vi "Open EXE or VI.vi"(8 "error in (no error)":errorcluster, 11 "Paths":string[](array[string])) -> (0 "error out":errorcluster)   [LabVIEW 2019, in "Control Experiment.lvclass"]
uses:
  Control Experiment.lvclass
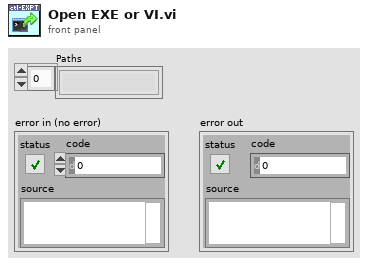
[diagram p1: front panel]
types:
  T1 = enum32{"Invalid", "Standard", "Closed", "Hidden", "Minimized", "Maximized"}
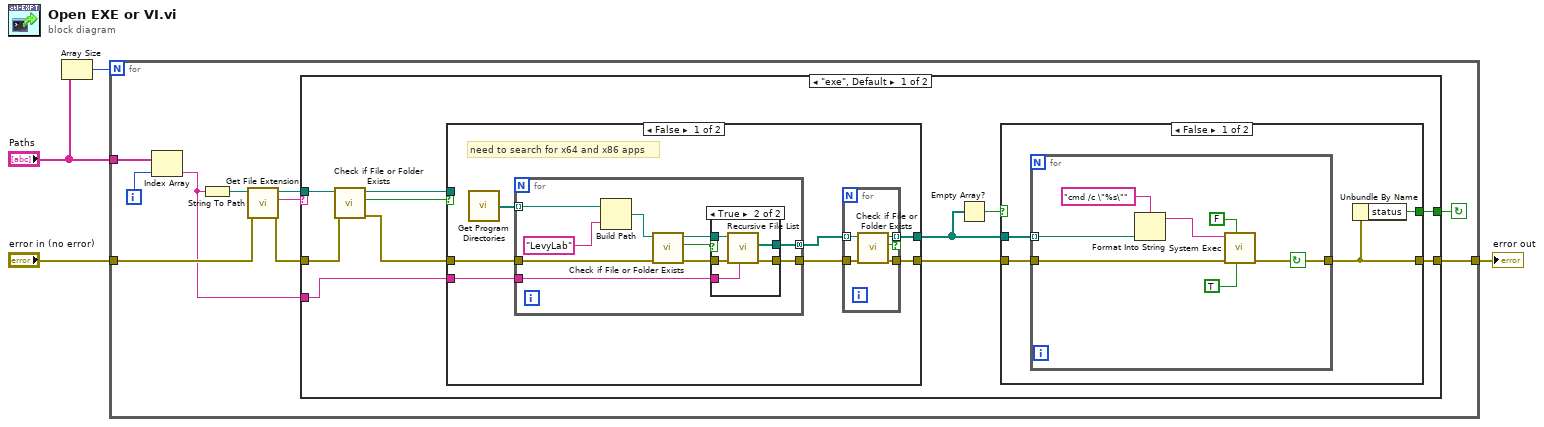
[diagram p0: block diagram]
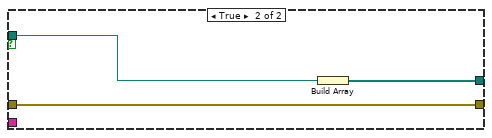
[diagram p3: hidden frame]
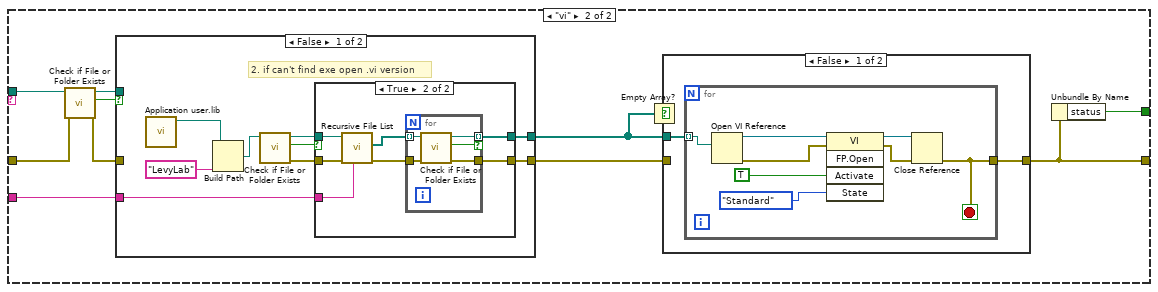
[diagram p5: hidden frame]
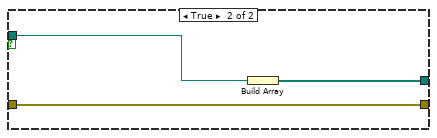
[diagram p7: hidden frame]
diagram:
  n1 = Array Size(array="Paths") -> (size(s)=w3:i32)
  n2 = for {
    N: w3 -> [_]
    tunnel: "error in (no error)" -> [w7]
    tunnel: [w14] -> w1
    tunnel: "Paths" -> [w12]
    i -> [w10]
    stop <- w13 continue-if-true
    n3 = Index Array(array=w12, index=w10) -> (element=w6:string)
    n4 = String To Path(string=w6) -> (path=w11:path)
    n5 = call <vilib>:"Get File Extension.vi"("error in (no error)"=w7, "file"=w11) -> ("error out"=w8:errorcluster, "lowercase file extension"=w9:string, "dup file"=w5:path)  [unwired: 5 in, 2 out]
    n6 = case shown="\"exe\", Default" w9 {
      tunnel: [w25 w80] -> w14
      tunnel: w8 -> [w18 w76]
      tunnel: [w23 w79] -> w13
      tunnel: w6 -> [w22 w78]
      tunnel: w5 -> [w21 w77]
      frame "exe", Default {
        n7 = call <vilib>:"Check if File or Folder Exists.vi"("error in (no error)"=w18, "path"=w21) -> ("error out"=w20:errorcluster, "file or folder exists?"=w19:bool, "dup path"=w17:path)  [unwired: 7 in]
        n8 = case shown="False" w19 {
          tunnel: w20 -> [w30 w56]
          tunnel: [w29 w56] -> w24
          tunnel: [w28 w55] -> w16
          tunnel: w22 -> [w27 _]
          tunnel: w17 -> [_ w54]
          frame False {
            # "need to search for x64 and x86 apps"
            n9 = call "Get Program Directories.vi"() -> ("Program Directories"=w32:path[])
            n10 = for {
              tunnel: w32 -> [w41] mode=indexing
              tunnel: w30 -> [w34]
              tunnel: [w40] -> w26
              tunnel: [w39] -> w31 mode=concatenating
              tunnel: w27 -> [w38]
              n11 = Build Path(base path=w41, name or relative path="LevyLab") -> (appended path=w37:path)
              n12 = call <vilib>:"Check if File or Folder Exists.vi"("error in (no error)"=w34, "path"=w37) -> ("error out"=w35:errorcluster, "file or folder exists?"=w33:bool, "dup path"=w36:path)  [unwired: 7 in]
              n13 = case shown="True" w33 {
                tunnel: [w43 w48] -> w40
                tunnel: [_ w47] -> w39
                tunnel: w38 -> [_ w46]
                tunnel: w36 -> [_ w45]
                tunnel: w35 -> [w43 w44]
                frame False {
                }
                frame True {
                  n14 = call <vilib>:"Recursive File List.vi"("pattern"=w46, "error in (no error)"=w44, "Folder Path"=w45) -> ("error out"=w48:errorcluster, "All Files in Dir"=w47:path[])  [unwired: 4 in, 3 out]
                }
              }
            }
            n15 = for {
              tunnel: w26 -> [w53]
              tunnel: w31 -> [w52] mode=indexing
              tunnel: [w51] -> w28 mode=indexing if=w49
              tunnel: [w50] -> w29
              n16 = call <vilib>:"Check if File or Folder Exists.vi"("error in (no error)"=w53, "path"=w52) -> ("error out"=w50:errorcluster, "file or folder exists?"=w49:bool, "dup path"=w51:path)  [unwired: 7 in]
            }
          }
          frame True {
            n17 = Build Array(w54) -> (w55:path[])
          }
        }
        n18 = Empty Array?(array=w16) -> (empty?=w15:bool)
        n19 = case shown="False" w15 {
          selector: w15 -> [_ w69]
          tunnel: [w58 w68] -> w25
          tunnel: w24 -> [w60 w68]
          tunnel: w16 -> [w59 _]
          tunnel: [w57 w69] -> w23
          frame False {
            n20 = for {
              tunnel: w59 -> [w62] mode=indexing
              tunnel: w60 -> [w64]
              tunnel: [w61] -> w58
              stop <- w61 continue-if-true
              n21 = Format Into String(format string="cmd /c \"%s\"", w62) -> (resulting string=w67:string)  [unwired: 2 in, 1 out]
              n22 = call <vilib>:"System Exec.vi"("run minimized? (F)"=TRUE, "wait until completion? (T)"=FALSE, "error in (no error)"=w64, "command line"=w67) -> ("error out"=w61:errorcluster)  [unwired: 4 in, 3 out]
            }
            n23 = Unbundle By Name(w58) -> ("status"=w57:bool)
          }
          frame True {
          }
        }
      }
      frame "vi" {
        n24 = call <vilib>:"Check if File or Folder Exists.vi"("error in (no error)"=w76, "path"=w77) -> ("error out"=w71:errorcluster, "file or folder exists?"=w70:bool, "dup path"=w72:path)  [unwired: 7 in]
        n25 = case shown="False" w70 {
          tunnel: [w88 w104] -> w74
          tunnel: [w87 w103] -> w73
          tunnel: w78 -> [w86 _]
          tunnel: w72 -> [_ w105]
          tunnel: w71 -> [_ w103]
          frame False {
            # "2. if can't find exe open .vi version"
            n26 = call "Application user.lib.vi"() -> ("path out"=w85:path)  [unwired: 10 in, 1 out]
            n27 = Build Path(base path=w85, name or relative path="LevyLab") -> (appended path=w84:path)
            n28 = call <vilib>:"Check if File or Folder Exists.vi"("path"=w84) -> ("error out"=w81:errorcluster, "file or folder exists?"=w82:bool, "dup path"=w83:path)  [unwired: 8 in]
            n29 = case shown="True" w82 {
              tunnel: [_ w97] -> w88
              tunnel: [w90 w96] -> w87
              tunnel: w86 -> [_ w95]
              tunnel: w83 -> [_ w93]
              tunnel: w81 -> [w90 w92]
              frame False {
              }
              frame True {
                n30 = call <vilib>:"Recursive File List.vi"("pattern"=w95, "error in (no error)"=w92, "Folder Path"=w93) -> ("error out"=w91:errorcluster, "All Files in Dir"=w94:path[])  [unwired: 4 in, 3 out]
                n31 = for {
                  tunnel: w91 -> [w102]
                  tunnel: w94 -> [w101] mode=indexing
                  tunnel: [w100] -> w97 mode=indexing if=w98
                  tunnel: [w99] -> w96
                  n32 = call <vilib>:"Check if File or Folder Exists.vi"("error in (no error)"=w102, "path"=w101) -> ("error out"=w99:errorcluster, "file or folder exists?"=w98:bool, "dup path"=w100:path)  [unwired: 7 in]
                }
              }
            }
          }
          frame True {
            n33 = Build Array(w105) -> (w104:path[])
          }
        }
        n34 = Empty Array?(array=w74) -> (empty?=w75:bool)
        n35 = case shown="False" w75 {
          tunnel: w74 -> [w107 _]
          tunnel: [w106 w116] -> w80
          tunnel: w73 -> [_ w116]
          frame False {
            n36 = for {
              tunnel: w107 -> [w108] mode=indexing
              tunnel: [w109] -> w106
              stop <- w109 stop-if-true
              n37 = Open VI Reference(vi path=w108) -> (vi reference=w110:refnum<vi>, error out=w115:errorcluster)  [unwired: 5 in]
              n38 = invoke class="VI" method="FP.Open"(reference=w110, error in=w115, "Activate"=TRUE ("Activate?"), "State"=T1."Standard") -> (reference out=w111:refnum<vi>, error out=w112:errorcluster)  [unwired: 1 in, 3 out]
              n39 = Close Reference(reference=w111, error in (no error)=w112) -> (error out=w109:errorcluster)
            }
          }
          frame True {
          }
        }
        n40 = Unbundle By Name(w80) -> ("status"=w79:bool)
      }
    }
  }
  "error out" <- w1
